vi "Kinesis - KDC101 - Build Device List.vi"() -> ()   [LabVIEW 2012]
uses:
  U:/Kinesis LabVIEW Website Examples/Thorlabs.MotionControl.DeviceManagerCLI.dll
  Thorlabs.MotionControl.DeviceManagerCLI.dll
  U:/Kinesis LabVIEW Website Examples/Thorlabs.MotionControl.Controls.dll
  Thorlabs.MotionControl.Controls.dll
panel:
  in  "?":bool
  in  "?":bool
  out "Selected Device":string
  out "Select Device":string[](array[string])
  in  "KCubeDCServoControl":refnum<k24>(container)
  # "Notes:"
  # "- Ensure that the appropriate .DLLs are copied into your Project Folder. Check that the correct bit type are used depending on your version of LabVIEW\ni.e. 32-bit or 64-bit.\n\n\n\n\n\n\n\n\n\n\n\n\n\n\n- Open the example VI through the LabVIEW Project Explorer to correctly load the User Interface from Thorlabs.MotionControl.Controls.dll."
  # "Description: This VI will enable you to search for & connect to your required controller. The VI will build a list of connected devices & wait until the user has selected the serialised device to control. This VI is currently setup to connect to a KDC101 & so a device with a prefix \"27***\" should be selected to successfully connect the device. Alternatively, you are able to change the device by inserting a different controller into the .NET Container. \n\nInstructions: \n1) Connect your KDC101 device to your PC & power the device, ensuring your stage/actutator is connected. For full device setup,  refer to the device product manual.\n2) Click 'Run' in the LabVIEW Toolbar.\n3) Scroll for your chosen device in the 'Select Device' array & then click 'SELECT DEVICE'\n4) To end the VI, click 'END'"
  # "Scroll Here to Select Device."
  # "Connected Device"
  # "Example Image of .NET Controller - VI opened via Project Explorer/ not opened via Project Explorer"
  # "VI Not Opened via Project Explorer"
  # "VI Opened via Project Explorer"
  # "Note: Right-click the .NET Container > 'Insert .NET Control' to change the Device Type."
  # "- To explore the range of methods available, please visit the .NET API, included with your Kinesis software.\n\n- For tips on building your own VIs with Thorlabs Motion Control Hardware, please see our LabVIEW Guide here.\nhttps://www.thorlabs.com/newgrouppage9.cfm?objectgroup_id=10285"
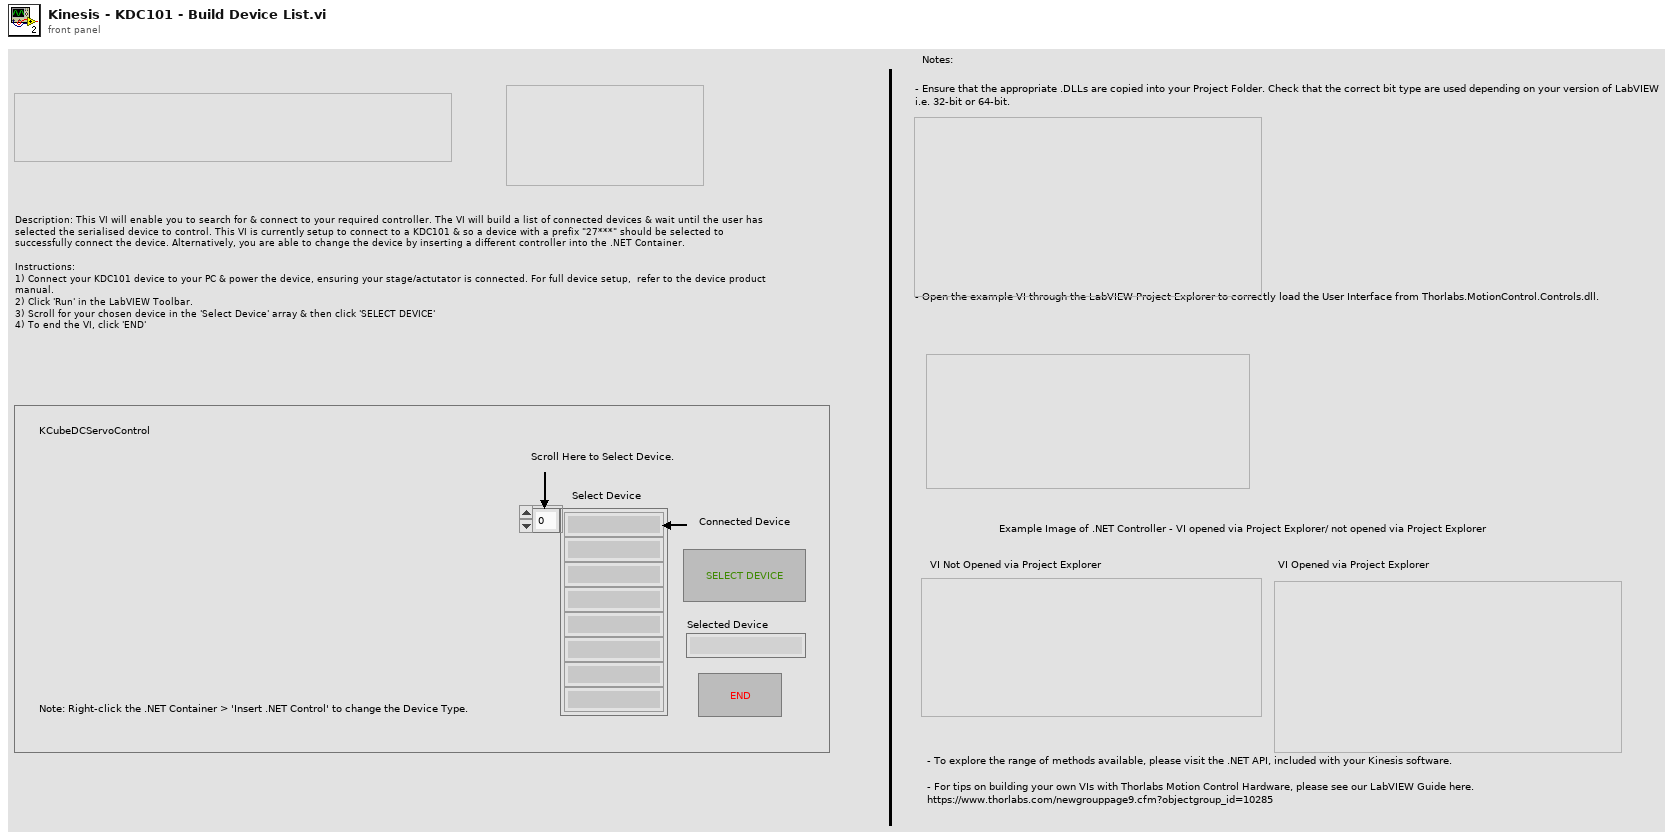
[diagram p1: front panel]
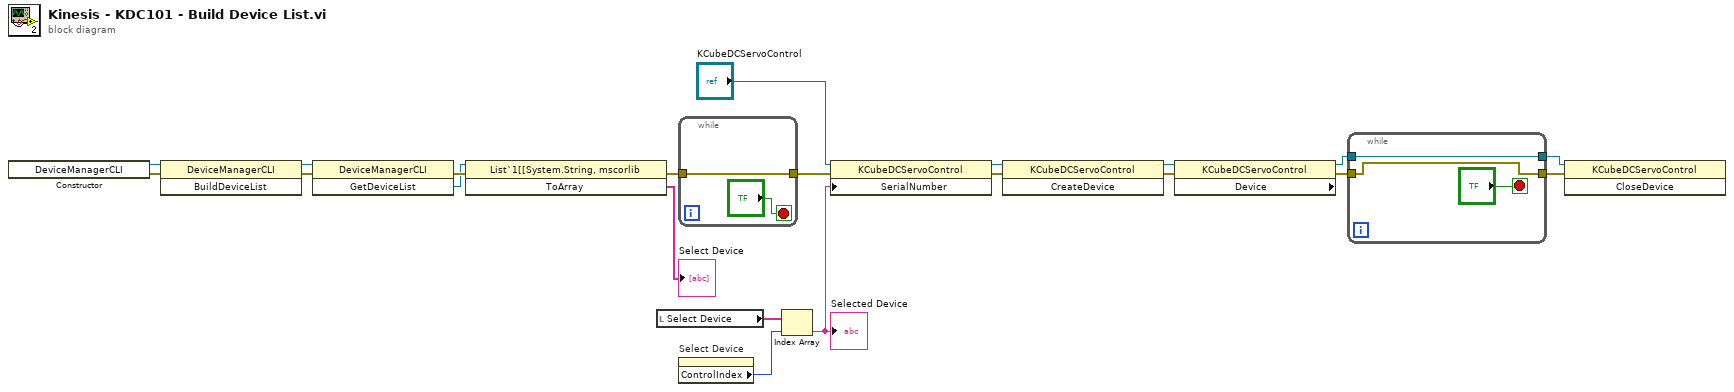
[diagram p0: block diagram]
diagram:
  n1 = constructor class="DeviceManagerCLI"() -> (reference out=w15:refnum<k24>, error out=w19:errorcluster)  [unwired: 3 in, 1 out]
  n2 = invoke class="DeviceManagerCLI" method="BuildDeviceList"(reference=w15, error in=w19) -> (reference out=w16:refnum<k24>, error out=w20:errorcluster)  [unwired: 1 in, 1 out]
  n3 = invoke class="DeviceManagerCLI" method="GetDeviceList"(reference=w16, error in=w20) -> (error out=w21:errorcluster, "GetDeviceList"=w17:refnum<k24>)  [unwired: 1 in, 1 out]
  n4 = invoke class="List`1[[System.String, mscorlib" method="ToArray"(reference=w17, error in=w21) -> (error out=w14:errorcluster, "ToArray"=→"Select Device":string[])  [unwired: 1 in, 1 out]
  n5 = local read "Select Device"() -> (w9:string[])
  n6 = while {
    tunnel: [w22] -> w11
    tunnel: w14 -> [w22]
    stop <- "?" stop-if-true
  }
  n7 = property on="Select Device" class="Arr (strict)"() -> ("ControlIndex"=w10:i32)  [unwired: 2 in, 2 out]
  n8 = Index Array(array=w9, index=w10) -> (element=w4:string)
  "Selected Device" <- w4
  n9 = property class="KCubeDCServoControl"(reference="KCubeDCServoControl", error in=w11, "SerialNumber"=w4) -> (reference out=w6:refnum<k24>, error out=w12:errorcluster)
  n10 = invoke class="KCubeDCServoControl" method="CreateDevice"(reference=w6, error in=w12) -> (reference out=w7:refnum<k24>, error out=w13:errorcluster)  [unwired: 1 in, 1 out]
  n11 = property class="KCubeDCServoControl" props=["Device"](reference=w7, error in=w13) -> (reference out=w8:refnum<k24>, error out=w3:errorcluster)  [unwired: 1 out]
  n12 = while {
    tunnel: [w26] -> w2
    tunnel: w8 -> [w26]
    tunnel: w3 -> [w24]
    tunnel: [w24] -> w1
    stop <- "?" stop-if-true
  }
  n13 = invoke class="KCubeDCServoControl" method="CloseDevice"(reference=w2, error in=w1) -> ()  [unwired: 1 in, 3 out]
